vi "BwCoeffMultiChanTemplate.vi"(0 "cutoff":dbl=2.0 format="%#_6p", 9 "sample rate":dbl=50000.0 format="%#_6p", 11 "error in (no error)":errorcluster, 12 "channel index":u16) -> (4 "configuration":T1, 15 "error out":errorcluster)   [LabVIEW 2020, in "NI_FpgaMspHost.lvlib"]
doc: "This VI designs a Butterworth filter, then quantizes and formats the coefficients into 32-bit integers for use by the Butterworth Filter VI on the FPGA.\n\nThe user is responsible for ensuring that the configuration is valid. The following restrictions apply:\nCutoff frequency must meet Nyquist criterion.\nMultichannel filters are restricted to 2nd order.\nFilter order and type cannot be changed at run-time."
uses:
  <vilib>/rvi/Analysis/host/Public/NI_FpgaMspHost.lvlib
  <vilib>/rvi/Analysis/host/Butterworth/config/Butterworth Filter Order.ctl
  <vilib>/rvi/Analysis/host/Butterworth/config/Butterworth Filter Type.ctl
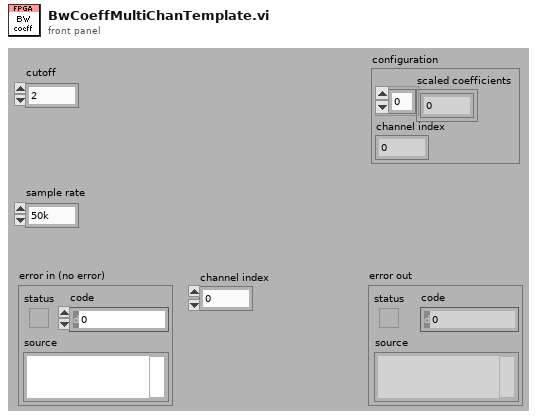
[diagram p1: front panel]
types:
  T1 = cluster{"scaled coefficients":i32[], "channel index":u16}
  T2 = typedef "NI_FpgaMspHost.lvlib/Butterworth Filter Type.ctl" = u16
  T3 = typedef "NI_FpgaMspHost.lvlib/Butterworth Filter Order.ctl" = i32
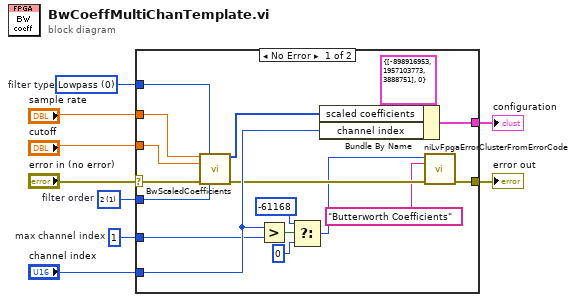
[diagram p0: block diagram]
diagram:
  w3 = T2 0 items=["Lowpass", "Highpass"]  # filter type
  w2 = T3 1 items=["1", "2", "4"]  # filter order
  w1 = u16 1  # max channel index
  n1 = case shown="No Error" "error in (no error)" {
    selector: "error in (no error)" -> [w17 w27]
    tunnel: "sample rate" -> [w26 _]
    tunnel: "cutoff" -> [w25 _]
    tunnel: [w22 _] -> w7
    tunnel: "channel index" -> [w20 _]
    tunnel: [w11 w27] -> w5
    tunnel: w3 -> [w16 _]
    tunnel: w2 -> [w15 _]
    tunnel: w1 -> [w14 _]
    frame No Error {
      n2 = call <vilib>:"BwScaledCoefficients.vi"("sample rate (S/s)"=w26, "filter type"=w16, "cutoff frequency (Hz)"=w25, "error in (no error)"=w17, "filter order"=w15) -> ("scaled coefficients"=w23:i32[], "error out"=w13:errorcluster)  [unwired: 9 out]
      n3 = Greater?(x=w20, y=w14) -> (0:w21:bool)
      n4 = Select(t=-61168, s=w21, f=0 ("Error Code")) -> (s? t:f=w12:i32)
      n5 = Bundle By Name(cluster=T1 {"scaled coefficients"=[-898916953, 1957103773, 3888751], "channel index"=0} ("scaled coefficients"), "scaled coefficients"=w23, "channel index"=w20) -> (w22:T1)
      n6 = call <vilib>:"niLvFpgaErrorClusterFromErrorCode.vi"("error code"=w12, "function name"="Butterworth Coefficients" ("subVI name"), "error in"=w13) -> ("error out"=w11:errorcluster)  [unwired: 4 in, 8 out]
    }
    frame Error {
    }
  }
  "error out" <- w5
  "configuration" <- w7
